vi "练习2：自动扫频.vi"   [LabVIEW 2021]
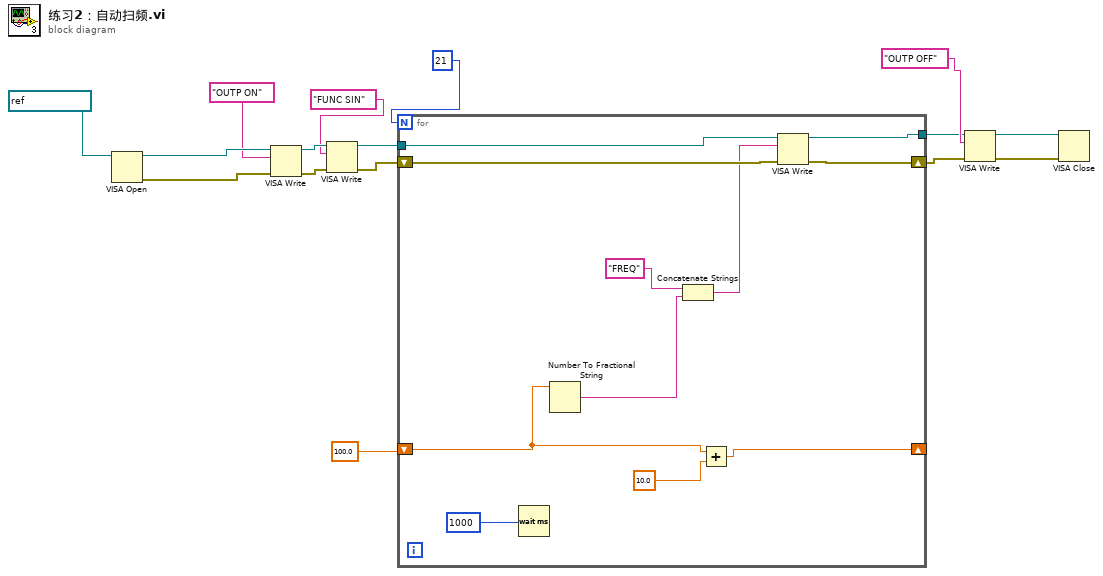
[diagram p0: block diagram]
diagram:
  n1 = VISA Open(VISA resource name=refnum<visa-resource-name> "DG1022U") -> (VISA resource name=w14:refnum<visa-resource-name>, error out=w16:errorcluster)  [unwired: 4 in]
  n2 = VISA Write(VISA resource name=w14, write buffer="OUTP ON", error in (no error)=w16) -> (VISA resource name out=w9:refnum<visa-resource-name>, error out=w8:errorcluster)  [unwired: 1 out]
  n3 = VISA Write(VISA resource name=w9, write buffer="FUNC SIN", error in (no error)=w8) -> (VISA resource name out=w3:refnum<visa-resource-name>, error out=w5:errorcluster)  [unwired: 1 out]
  n4 = for {
    N: 21 -> [_]
    shift-right: [w24] -> w4
    shift-left: w5 -> [w25]
    tunnel: w3 -> [w27]
    tunnel: [w26] -> w2
    shift-right: [w20] -> _
    shift-left: 100.0 -> [w22]
    n5 = Wait (ms)(milliseconds to wait=1000) -> ()  [unwired: 1 out]
    n6 = Number To Fractional String(number=w22) -> (F-format string=w19:string)  [unwired: 3 in]
    n7 = Concatenate Strings("FREQ", w19) -> (w18:string)
    n8 = Add(x=w22, y=10.0) -> (x+y=w20:dbl)
    n9 = VISA Write(VISA resource name=w27, write buffer=w18, error in (no error)=w25) -> (VISA resource name out=w26:refnum<visa-resource-name>, error out=w24:errorcluster)  [unwired: 1 out]
  }
  n10 = VISA Write(VISA resource name=w2, write buffer="OUTP OFF", error in (no error)=w4) -> (VISA resource name out=w13:refnum<visa-resource-name>, error out=w15:errorcluster)  [unwired: 1 out]
  n11 = VISA Close(VISA resource name=w13, error in (no error)=w15) -> ()  [unwired: 1 out]
